vi "uDAQserver.vi"(10 "Rate":T1(ring)=enum."500Hz", 11 "FS Range":sgl=0.1445092) -> ()   [LabVIEW 2017]
panel:
  out "Status":string
  in  "Stop Button":bool
  out "error out":errorcluster
  in  "NextArrayBuf":i32
  in  "Residual Buffer":string[](array[string])
  in  "RawBuffer":string[](array[string])
  in  "Process":string
  in  "Byte Count":u32
  in  "RX Buffer":string
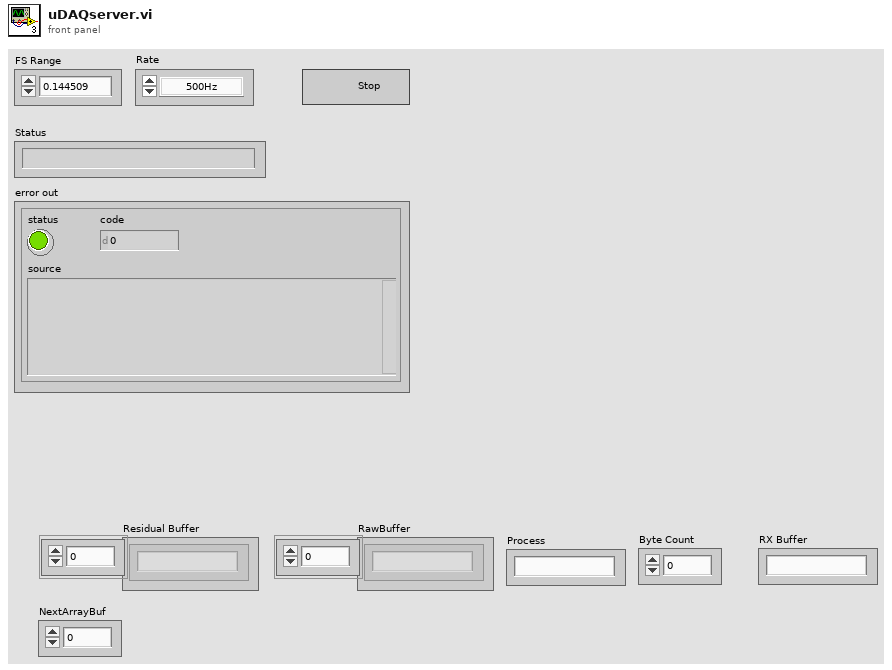
[diagram p1: front panel]
types:
  T1 = enum16{"Off", "1Hz", "5Hz", "10Hz", "20Hz", "25Hz", "50Hz", "100Hz", "150Hz", "200Hz", "225Hz", "312Hz", "400Hz", "500Hz", "625Hz", "1000Hz"}
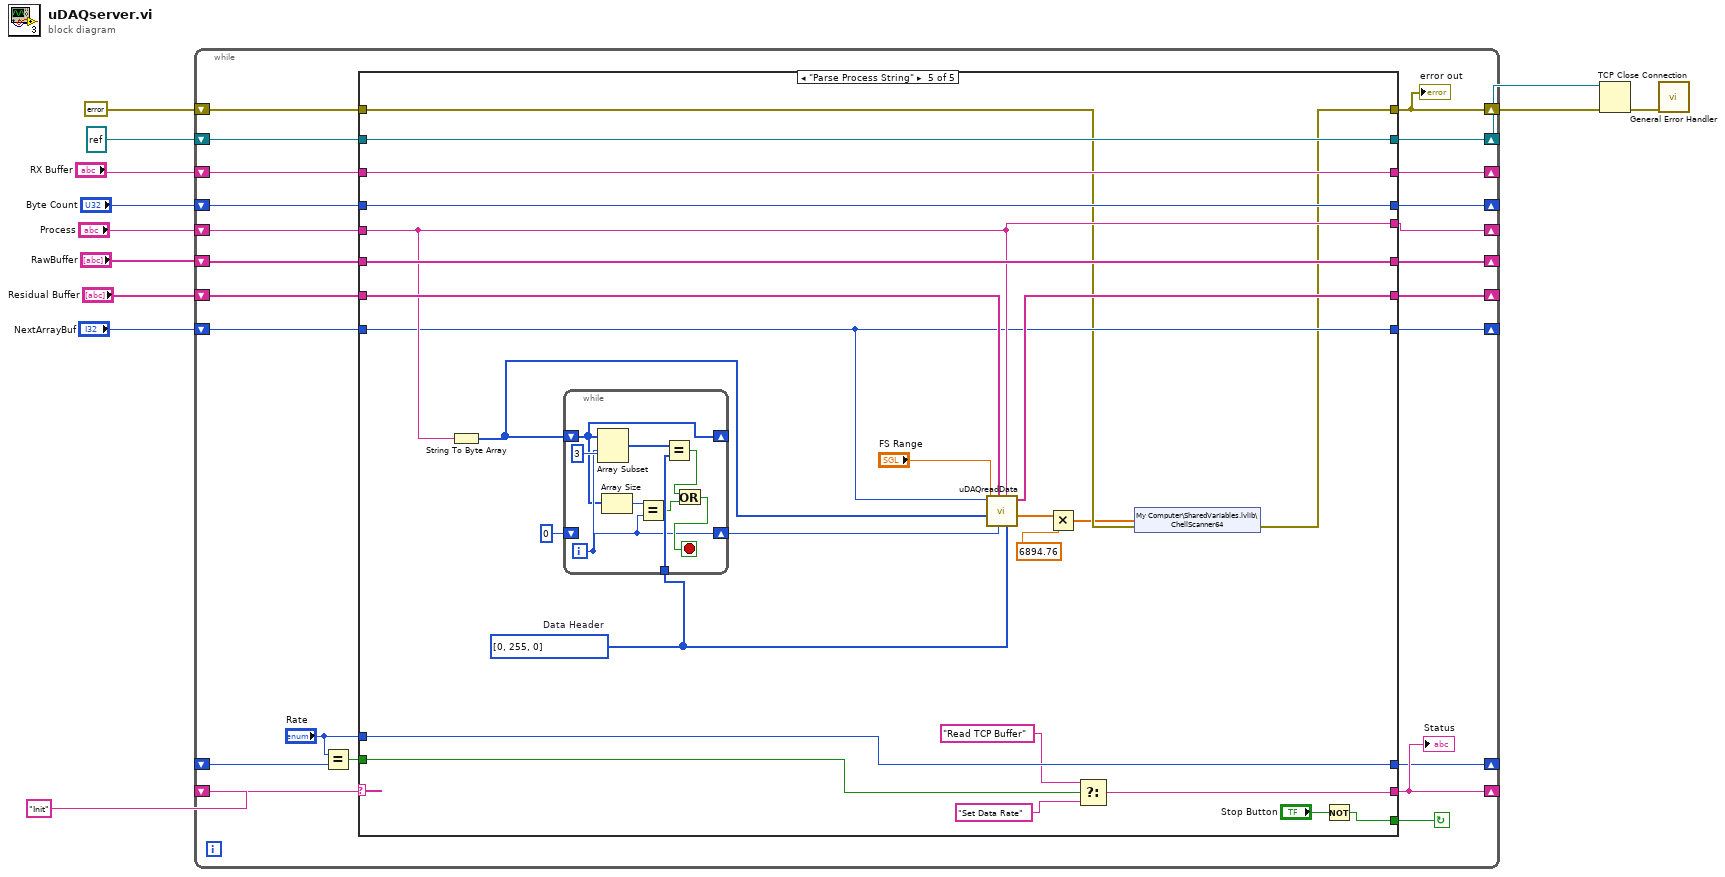
[diagram p0: block diagram]
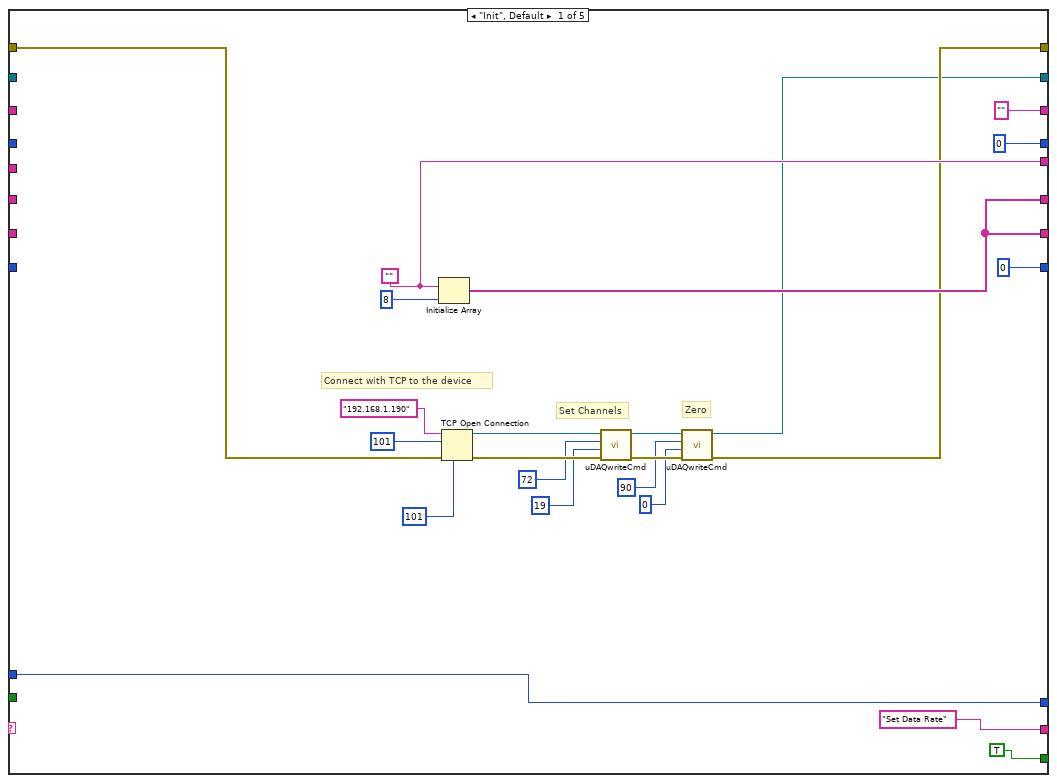
[diagram p2: hidden frame]
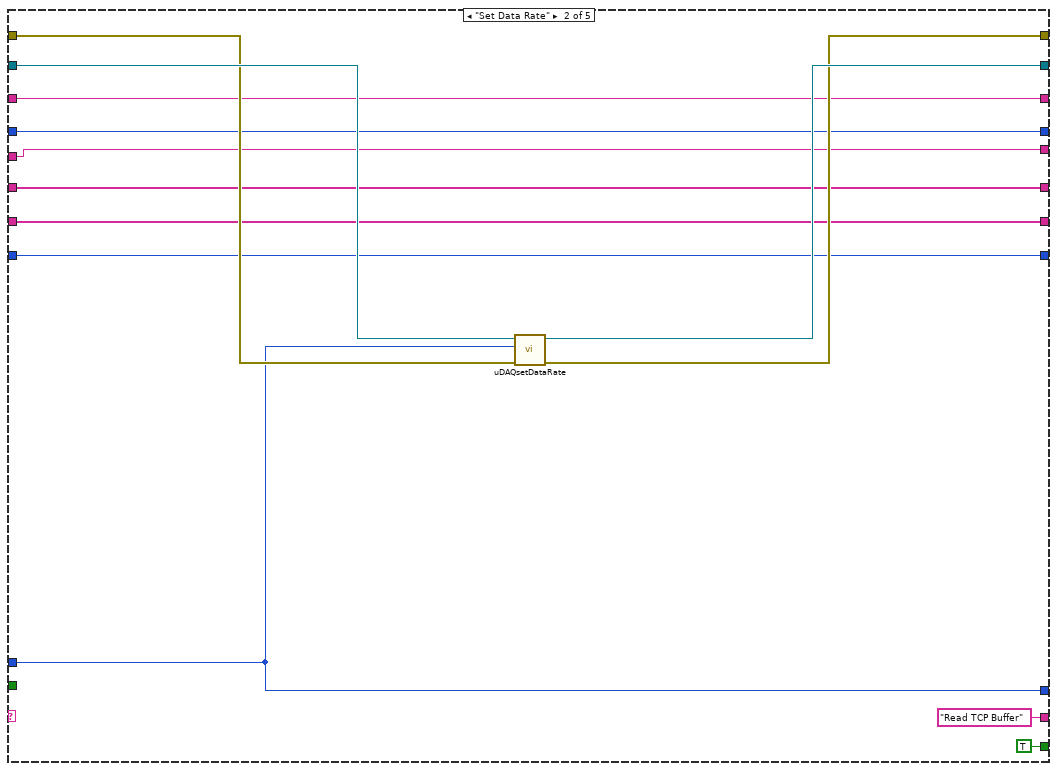
[diagram p3: hidden frame]
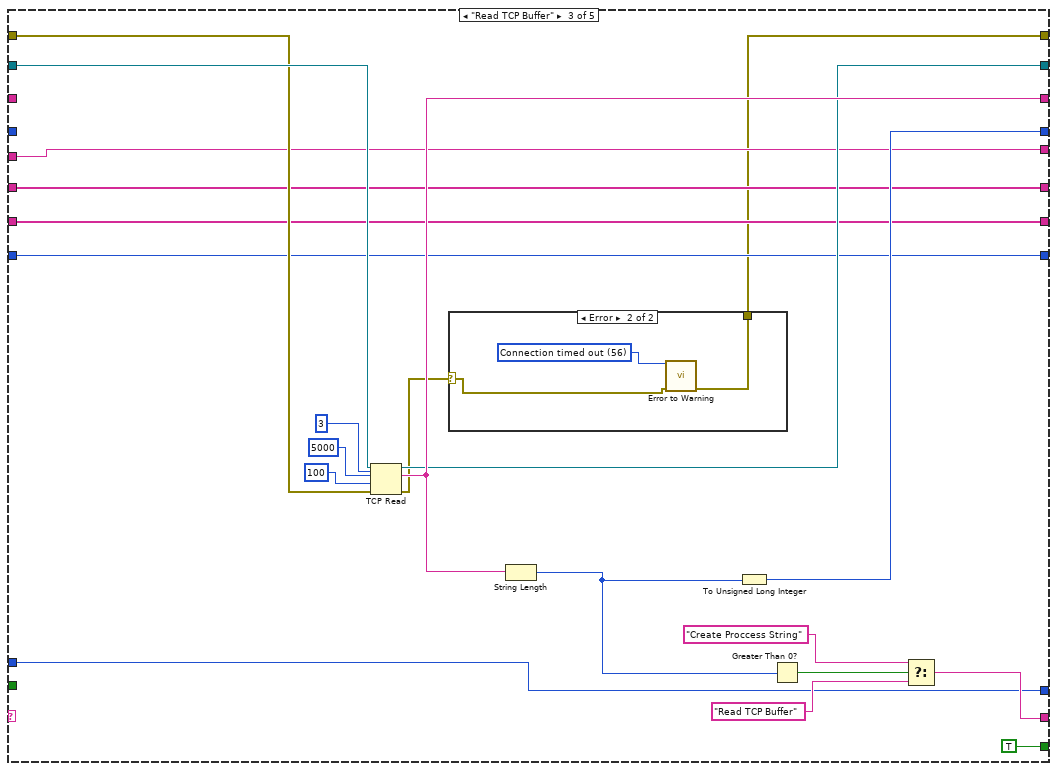
[diagram p4: hidden frame]
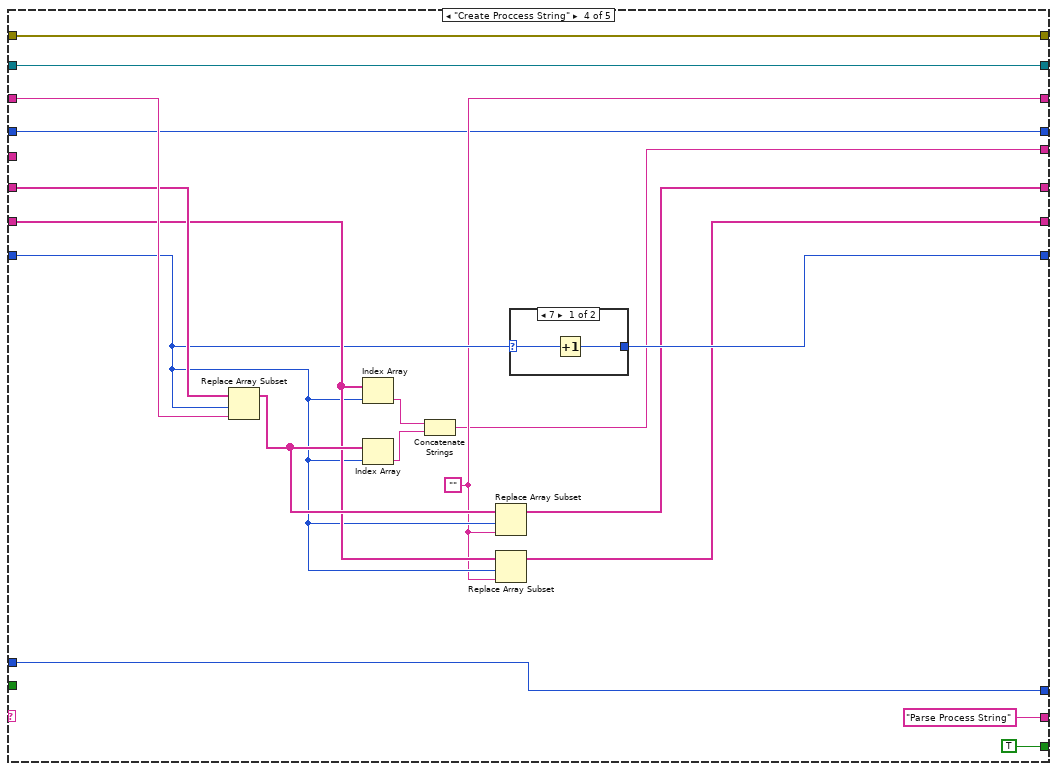
[diagram p6: hidden frame]
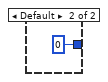
[diagram p7: hidden frame]
diagram:
  n1 = while {
    shift-right: [w18] -> w1
    shift-left: errorcluster {"status"=FALSE, "code"=0, "source"=""} ("error in (no error)") -> [w35]
    shift-right: [w33] -> _
    shift-left: "RX Buffer" -> [w34]
    shift-right: [w31] -> _
    shift-left: "Byte Count" -> [w32]
    shift-right: [w30] -> _
    shift-left: "Init" -> [w29]
    shift-right: [w28] -> w2
    shift-left: refnum<k5> refnum ("connection ID out") -> [w27]
    shift-right: [w26] -> _
    shift-left: "Process" -> [w25]
    shift-right: [w24] -> _
    shift-left: "RawBuffer" -> [w22]
    shift-right: [w23] -> _
    shift-left: "Residual Buffer" -> [w21]
    shift-right: [w19] -> _
    shift-left: "NextArrayBuf" -> [w20]
    shift-right: [w16] -> _
    shift-left: _ -> [w14]
    stop <- w17 continue-if-true
    n2 = Equal?(x="Rate", y=w14) -> (x = y?=w13:bool)
    n3 = case shown="\"Parse Process String\"" w29 {
      tunnel: w35 -> [w55 w66 w87 w102 w129]
      tunnel: [w38 w67 w73 w102 w128] -> w18
      tunnel: w34 -> [_ w65 _ w114 w134]
      tunnel: ["" ("RX Buffer") w65 w86 w106 w134] -> w33
      tunnel: w32 -> [_ w64 _ w100 w133]
      tunnel: [u32 0 ("Byte Count") w64 w85 w100 w133] -> w31
      tunnel: ["Set Data Rate" ("RX Buffer") "Read TCP Buffer" ("RX Buffer") w79 "Parse Process String" ("RX Buffer") w123] -> w30
      tunnel: [TRUE TRUE TRUE TRUE w126] -> w17
      tunnel: [w37 w68 w84 w103 w135] -> w28
      tunnel: w27 -> [_ w69 w88 w103 w135]
      tunnel: [w49 w63 w76 w101 w131] -> w26
      tunnel: w25 -> [_ w63 w76 _ w131]
      tunnel: [w48 w62 w77 w105 w132] -> w24
      tunnel: [w48 w61 w78 w104 w137] -> w23
      tunnel: w22 -> [_ w62 w77 w113 w132]
      tunnel: w21 -> [_ w61 w78 w108 w138]
      tunnel: w20 -> [_ w60 w75 w107 w130]
      tunnel: [0 w60 w75 w110 w130] -> w19
      tunnel: "Rate" -> [w36 w59 w72 w97 w125]
      tunnel: [w36 w59 w72 w97 w125] -> w16
      tunnel: w13 -> [_ _ _ _ w124]
      frame "Init", Default {
        w49 = ""
        # "Zero"
        # "Set Channels"
        # "Connect with TCP to the device"
        n4 = Initialize Array(w49, 8) -> (w48:string[])
        n5 = TCP Open Connection(address="192.168.1.190", remote port or service name=u16 101, local port=u16 101 ("local port (0)"), error in (no error)=w55) -> (connection ID=w46:refnum<k5>, error out=w45:errorcluster)  [unwired: 1 in]
        n6 = call "uDAQwriteCmd.vi"("error in (no error)"=w45, "ParamByte"=u8 19, "CmdByte"=u8 72, "connection ID"=w46) -> ("error out"=w41:errorcluster, "connection ID out"=w42:refnum<k5>)  [unwired: 6 in]
        n7 = call "uDAQwriteCmd.vi"("error in (no error)"=w41, "ParamByte"=u8 0, "CmdByte"=u8 90, "connection ID"=w42) -> ("error out"=w38:errorcluster, "connection ID out"=w37:refnum<k5>)  [unwired: 6 in]
      }
      frame "Set Data Rate" {
        n8 = call "uDAQsetDataRate.vi"("error in (no error)"=w66, "Menu Ring"=w59, "connection ID"=w69) -> ("error out"=w67:errorcluster, "connection ID out"=w68:refnum<k5>)  [unwired: 7 in]
      }
      frame "Read TCP Buffer" {
        n9 = TCP Read(connection ID=w88, bytes to read=5000, error in (no error)=w87, 7:u8 3, 9:100) -> (connection ID out=w84:refnum<k5>, data out=w86:string, error out=w74:errorcluster)
        n10 = case shown="Error" w74 {
          selector: w74 -> [w93 w95]
          tunnel: [w93 w94] -> w73
          frame No Error {
          }
          frame Error {
            w96 = 56 items=["No Error", "Argument Error", "Memory Full", "Out of Zone", "End of File", "File Already Open", "Generic File IO Error", "File Not Found", "File Permission Error", "Disk Full", "Duplicate Path", "Too Many Files Open", "Not Enabled", "Resource File Not Found", "Cannot Add Resource", "Resource Not Found", "Image Not Found", "Image Memory Error", "Pen Does Not Exist", "Config Bad Type", "Config Token Not Found", "Config Parse Error", "Config Memory Error", "Bad External Code Format", "Bad External Code Offset", "External Code Not Present", "Null Window", "Destroy Window Mixup", "Null Menu", "Print Aborted", "Bad Print Record", "Print Driver Error", "Windows Error During Print", "Memory Error During Print", "Print Dialog Error", "Generic Print Error", "Invalid Device Refnum", "Device Not Found", "Device Parameter Error", "Device Unit Error", "Can't Open Device", "Device Call Aborted", "Generic Error", "Cancelled By User", "Object ID Too Low", "Object ID Too High", "Object Not In Heap", "Unknown Heap", "Bad DefProc ID", "DefProc Not In Table", "Message Out Of Range", "Null Method", "Unknown Message", "Manager Call Not Supported", "Bad address", "Connection In progress", "Connection timed out", "Connection is already in progress", "Network attribute not supported", "Network error", "Address in use", "System out of memory", "Connection aborted", "Connection refused", "Connection is not connected", "Connection is already connected", "Connection closed", "Initialize error (interapplication manager)", "Bad occurrence", "Wait on unbound occurrence handler", "Occurrence queue overflow", "Bad path", "Semaphore not signaled", "Unrecognized type (interapplication manager)"] ("1st Error to Convert")
            n11 = call <vilib>:"Error to Warning.vi"("1st Error to Convert"=w96, "error in"=w95) -> ("warning out"=w94:errorcluster)  [unwired: 13 in]
          }
        }
        n12 = String Length(string=w86) -> (length=w83:i32)
        n13 = To Unsigned Long Integer(number=w83) -> (unsigned 32bit integer=w85:u32)
        n14 = Greater Than 0?(x=w83) -> (x > 0?=w82:bool)
        n15 = Select(t="Create Proccess String" ("RX Buffer"), s=w82, f="Read TCP Buffer" ("RX Buffer")) -> (s? t:f=w79:string)
      }
      frame "Create Proccess String" {
        w106 = ""
        n16 = Replace Array Subset(array=w113, new element=w114, index=w107) -> (w109:string[])
        n17 = Index Array(array=w108, index=w107) -> (element=w111:string)
        n18 = Index Array(array=w109, index=w107) -> (element=w112:string)
        n19 = Concatenate Strings(w111, w112) -> (w101:string)
        n20 = Replace Array Subset(array=w109, new element=w106, index=w107) -> (w105:string[])
        n21 = Replace Array Subset(array=w108, new element=w106, index=w107) -> (w104:string[])
        n22 = case shown="7" w107 {
          selector: w107 -> [w116 _]
          tunnel: [w115 0] -> w110
          frame 7 {
            n23 = Increment(x=w116) -> (x+1=w115:i32)
          }
          frame Default {
          }
        }
      }
      frame "Parse Process String" {
        w139 = u8[] [0, 255, 0]  # Data Header
        n24 = String To Byte Array(string=w131) -> (unsigned byte array=w140:u8[])
        n25 = while {
          tunnel: w139 -> [w148]
          shift-right: [w146] -> w141
          shift-left: 0 -> [_]
          shift-right: [w143] -> _
          shift-left: w140 -> [w143]
          i -> [w146]
          stop <- w149 stop-if-true
          n26 = Array Subset(array=w143, index=w146, length=3) -> (w150:u8[])
          n27 = Array Size(array=w143) -> (size(s)=w145:i32)
          n28 = Equal?(x=w145, y=w146) -> (x = y?=w144:bool)
          n29 = Equal?(x=w150, y=w148) -> (x = y?=w147:bool)
          n30 = Or(x=w147, y=w144) -> (x .or. y?=w149:bool)
        }
        n31 = call "uDAQreadData.vi"("Data Header"=w139, "Process"=w131, "DataStart"=w141, "Residual Buffer in"=w138, "ByteArray"=w140, "FS Range"="FS Range", "NextArrayBuf"=w130) -> ("Data"=w119:dbl[], "Residual Buffer out"=w137:string[])  [unwired: 3 in]
        n32 = Multiply(x=w119, y=6894.76) -> (x*y=w118:dbl[])
        n33 = Select(t="Read TCP Buffer" ("RX Buffer"), s=w124, f="Set Data Rate" ("RX Buffer")) -> (s? t:f=w123:string)
        n34 = shared-variable "My Computer\\SharedVariables.lvlib\\ChellScanner64"(w118, error in=w129) -> (error out=w128:errorcluster)
        n35 = Not(x="Stop Button") -> (.not. x?=w126:bool)
      }
    }
    "error out" <- w18
    "Status" <- w30
  }
  n36 = TCP Close Connection(connection ID=w2, error in (no error)=w1) -> (error out=w7:errorcluster)  [unwired: 1 in, 1 out]
  n37 = call <vilib>:"General Error Handler.vi"("error in (no error)"=w7) -> ()  [unwired: 10 in, 5 out]
